vi "Read Lock-in Configuration.vi"(8 "error in (no error)":errorcluster, 11 "Lock-in in":refnum<class "Lock-in.lvclass">) -> (0 "error out":errorcluster, 2 "Configuration":T1 {"Time constant" format="%#_6ps"; "Frequency" format="%#_6pHz"}, 3 "Lock-in out":refnum<class "Lock-in.lvclass">)   [LabVIEW 2015, in "Lock-in.lvclass"]
uses:
  Lock-in.lvclass
  NHMFL_Core/Libraries/Instruments/Instrument Driver/Lock-in Driver/Lock-in Configuration.ctl
  Measure_core/Measure Object/Measure Object.lvclass/Measure Object.ctl
  Measure_core/Measure Object/Read Configuration.vi
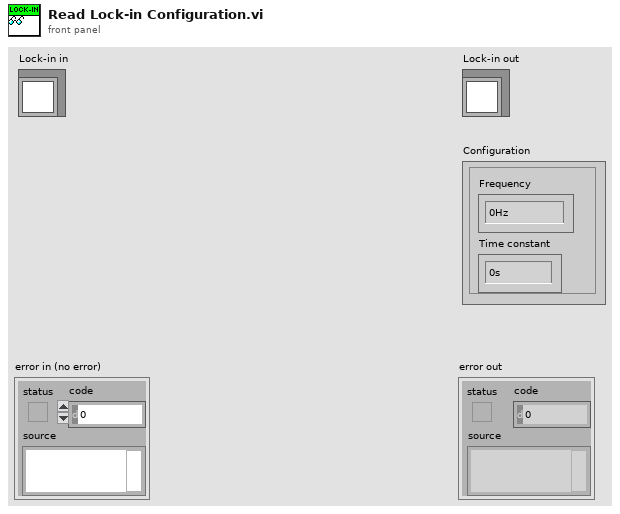
[diagram p1: front panel]
types:
  T1 = typedef "Lock-in Configuration.ctl" = cluster{"Frequency":dbl, "Time constant":dbl}
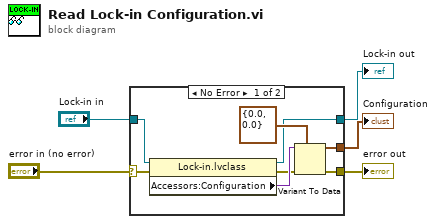
[diagram p0: block diagram]
diagram:
  n1 = case shown="No Error" "error in (no error)" {
    selector: "error in (no error)" -> [w7 w14]
    tunnel: [w12 w14] -> w4
    tunnel: [w10 w15] -> w2
    tunnel: "Lock-in in" -> [w13 w15]
    tunnel: [w8 _] -> w1
    frame No Error {
      n2 = property class="Lock-in.lvclass"(reference=w13, error in=w7) -> (reference out=w10:refnum<class "Lock-in.lvclass">, error out=w6:errorcluster, "Accessors:Configuration"=w9:variant)
      n3 = Variant To Data(error in=w6, type=T1 {"Frequency"=0.0, "Time constant"=0.0} ("Configuration"), Variant=w9) -> (data=w8:T1, error out=w12:errorcluster)
    }
    frame Error {
    }
  }
  "error out" <- w4
  "Lock-in out" <- w2
  "Configuration" <- w1
